vi "Intan_binary_to_uV.vi"(3 "2d ADC binary data":u16[][](array[numeric])) -> (1 "Scaled Data (uV)":dbl[][](array[numeric]))   [LabVIEW 2020]
doc: "Scales uint16 ADC data to physical units of uV. Input and output data arrays are Nchans x Nsamps (signals in rows)"
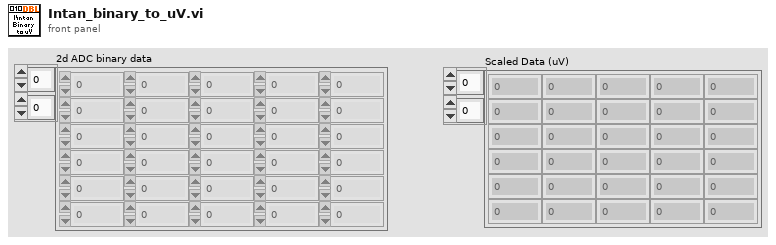
[diagram p1: front panel]
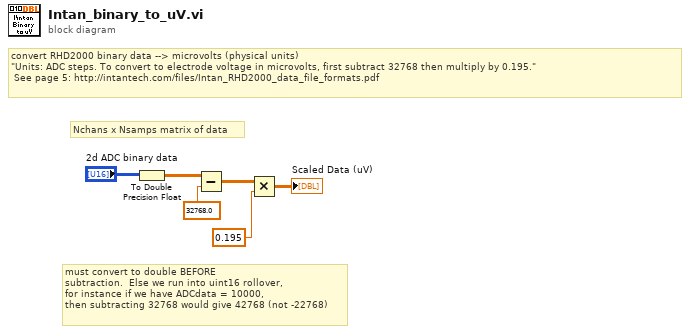
[diagram p0: block diagram]
diagram:
  # "must convert to double BEFORE \nsubtraction.  Else we run into uint16 rollover,\nfor instance if we have ADCdata = 10000, \nthen subtracting 32768 would give 42768 (not -22768)"
  # "convert RHD2000 binary data --> microvolts (physical units)\n\"Units: ADC steps. To convert to electrode voltage in microvolts, first subtract 32768 then multiply by 0.195.\"\n See page 5: http://intantech.com/files/Intan_RHD2000_data_file_formats.pdf"
  # "Nchans x Nsamps matrix of data"
  n1 = To Double Precision Float(number="2d ADC binary data") -> (double precision float=w1:dbl[][])
  n2 = Subtract(x=w1, y=32768.0) -> (x-y=w5:dbl[][])
  n3 = Multiply(x=w5, y=0.195) -> (x*y=→"Scaled Data (uV)":dbl[][])
